vi "U01_4_MultipleClients.vi"() -> ()   [LabVIEW 2015]
panel:
  in  "Salir":bool
  out "data out 2":string
  in  "mode (standard) 2":T1(ring)
  out "error out":errorcluster
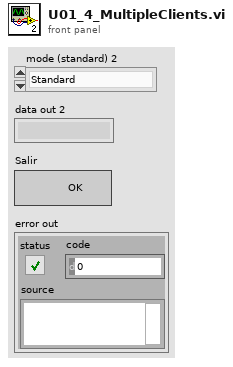
[diagram p1: front panel]
types:
  T1 = enum16{"Standard", "Buffered", "CRLF", "Immediate"}
  T2 = cluster{"connection ID":refnum<k5>, "service name":string, "port":u16}
  T3 = cluster{"Message":string, "ID":i32, "TCPCL":cluster{"connection ID":refnum<k5>, "service name":string, "port":u16}}
  T4 = cluster{string, "ID":i32, "TCPCL":cluster{"connection ID":refnum<k5>, "service name":string, "port":u16}}
  T5 = cluster{string, i32, "TCPCL":cluster{"connection ID":refnum<k5>, "service name":string, "port":u16}}
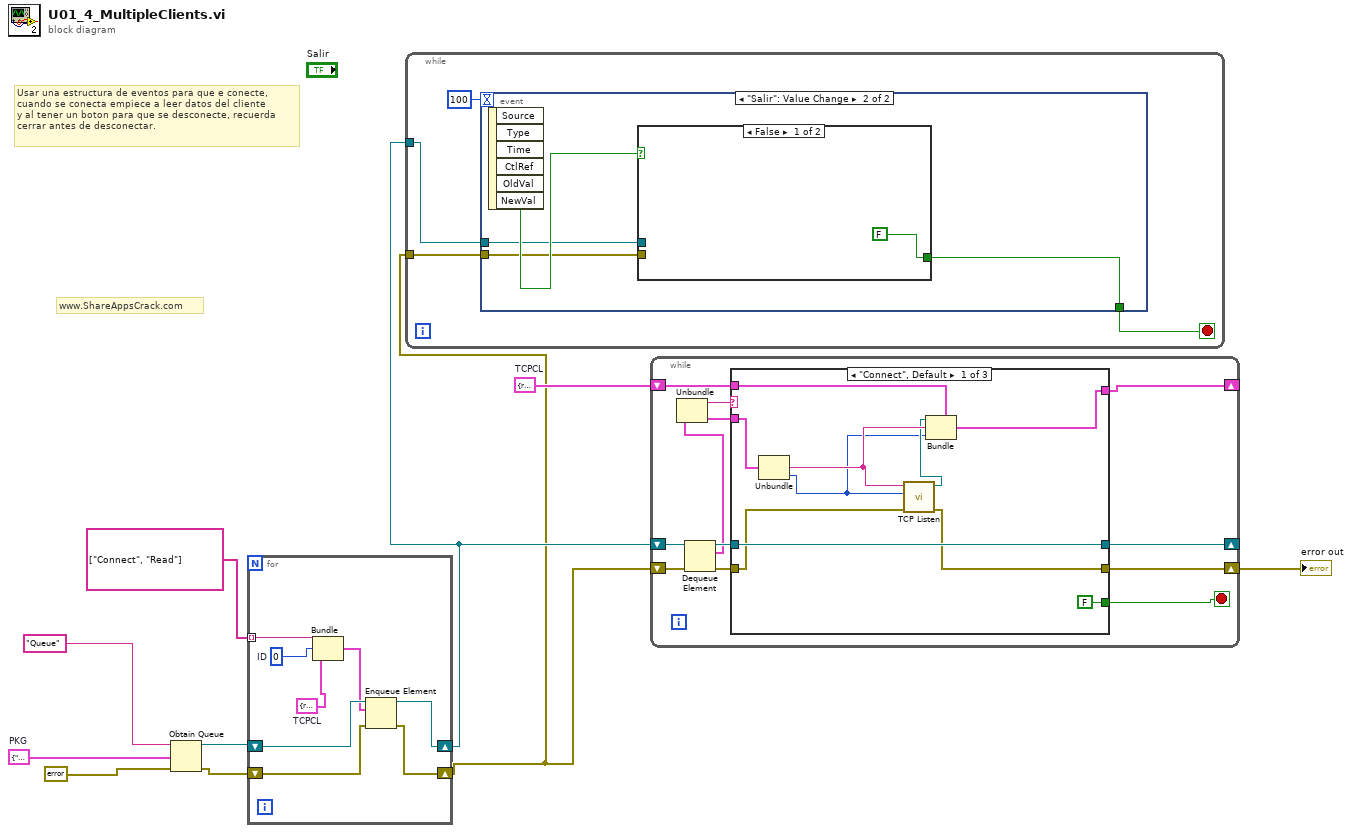
[diagram p0: block diagram]
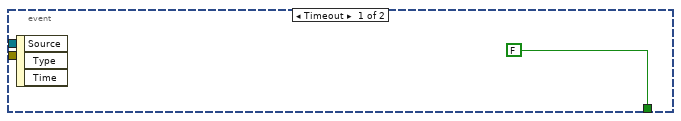
[diagram p2: hidden frame]
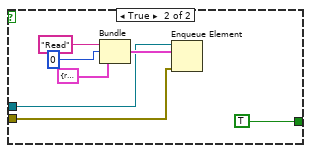
[diagram p3: hidden frame]
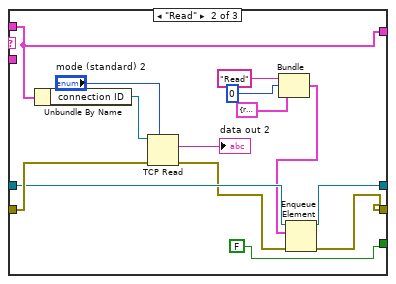
[diagram p4: hidden frame]
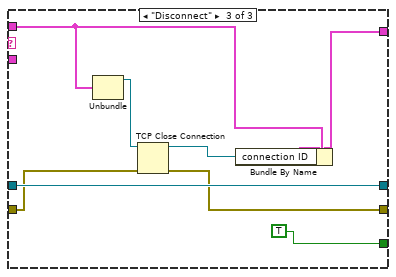
[diagram p5: hidden frame]
diagram:
  w3 = T2 {"connection ID"=refnum, "service name"="127.0.0.1", "port"=80}  # TCPCL
  w7 = T3 {"Message"="", "ID"=0, "TCPCL"={"connection ID"=refnum, "service name"="", "port"=0}}  # PKG
  # "Usar una estructura de eventos para que e conecte,\ncuando se conecta empiece a leer datos del cliente\ny al tener un boton para que se desconecte, recuerda \ncerrar antes de desconectar."
  # "www.ShareAppsCrack.com"
  n1 = Obtain Queue(name (unnamed)="Queue", element data type=w7, error in (no error)=errorcluster {"status"=FALSE, "code"=0, "source"=""}) -> (queue out=w6:refnum<queue>, error out=w5:errorcluster)  [unwired: 2 in, 1 out]
  n2 = for {
    shift-right: [w11] -> w2
    shift-left: w6 -> [w15]
    shift-right: [w12] -> w1
    shift-left: w5 -> [w13]
    tunnel: string[] ["Connect", "Read"] -> [w18] mode=indexing
    w16 = T2 {"connection ID"=refnum, "service name"="", "port"=0}  # TCPCL
    w17 = 0  # ID
    n3 = Bundle(w18, "ID"=w17, "TCPCL"=w16) -> (w14:T4)  [unwired: 1 in]
    n4 = Enqueue Element(queue=w15, element=w14, error in (no error)=w13) -> (queue out=w11:refnum<queue>, error out=w12:errorcluster)  [unwired: 1 in, 1 out]
  }
  n5 = while {
    tunnel: w2 -> [w21]
    tunnel: w1 -> [w20]
    stop <- w19 stop-if-true
    n6 = event shown="[1] \"Salir\": Value Change" {
      selector: _ -> [_ _]
      dyn-events: _ -> [_ _]
      timeout: 100 -> [_ _]
      tunnel: w21 -> [_ w26]
      tunnel: w20 -> [_ w25]
      tunnel: [FALSE w24] -> w19
      event Timeout {
        n7 = event-data() -> ()  [unwired: 1 in, 3 out]
      }
      event "Salir": Value Change {
        n8 = event-data() -> ("NewVal"=w27:bool)  [unwired: 1 in, 5 out]
        n9 = case shown="False" w27 {
          tunnel: w26 -> [_ w31]
          tunnel: w25 -> [_ w30]
          tunnel: [FALSE TRUE] -> w24
          frame False {
          }
          frame True {
            n10 = Bundle("Read", 0, "TCPCL"=T2 {"connection ID"=refnum, "service name"="127.0.0.1", "port"=80}) -> (w32:T5)  [unwired: 1 in]
            n11 = Enqueue Element(queue=w31, element=w32, error in (no error)=w30) -> ()  [unwired: 1 in, 3 out]
          }
        }
      }
    }
  }
  n12 = while {
    shift-right: [w46] -> w8
    shift-left: w1 -> [w42]
    shift-right: [w47] -> _
    shift-left: w2 -> [w44]
    shift-right: [w37] -> _
    shift-left: w3 -> [w36]
    stop <- w45 stop-if-true
    n13 = Dequeue Element(queue=w44, error in (no error)=w42) -> (queue out=w43:refnum<queue>, element=w40:T3, error out=w41:errorcluster)  [unwired: 1 in, 1 out]
    n14 = Unbundle(w40) -> ("Message"=w39:string, "TCPCL"=w38:T2)  [unwired: 1 out]
    n15 = case shown="\"Connect\", Default" w39 {
      tunnel: w41 -> [w56 w68 w78]
      tunnel: w43 -> [w57 w67 w79]
      tunnel: [w57 w66 w79] -> w47
      tunnel: [w55 w64 w77] -> w46
      tunnel: [FALSE ("status") FALSE TRUE] -> w45
      tunnel: w38 -> [w54 _ _]
      tunnel: [w48 w59 w74] -> w37
      tunnel: w36 -> [w52 w59 w75]
      frame "Connect", Default {
        n16 = Unbundle(w54) -> ("service name"=w51:string, "port"=w49:u16)  [unwired: 1 out]
        n17 = call <vilib>:"TCP Listen.vi"("error in (no error)"=w56, "port"=w49, "service name"=w51) -> ("error out"=w55:errorcluster, "connection ID"=w50:refnum<k5>)  [unwired: 4 in, 3 out]
        n18 = Bundle(cluster=w52, "connection ID"=w50, "service name"=w51, "port"=w49) -> (w48:T2)
      }
      frame "Read" {
        n19 = Unbundle By Name(w59) -> ("connection ID"=w71:refnum<k5>)
        n20 = TCP Read(connection ID=w71, error in (no error)=w68, 7:"mode (standard) 2") -> (data out=→"data out 2":string, error out=w65:errorcluster)  [unwired: 2 in, 1 out]
        n21 = Bundle("Read", 0, "TCPCL"=T2 {"connection ID"=refnum, "service name"="127.0.0.1", "port"=80}) -> (w60:T5)  [unwired: 1 in]
        n22 = Enqueue Element(queue=w67, element=w60, error in (no error)=w65) -> (queue out=w66:refnum<queue>, error out=w64:errorcluster)  [unwired: 1 in, 1 out]
      }
      frame "Disconnect" {
        n23 = Unbundle(w75) -> ("connection ID"=w76:refnum<k5>)  [unwired: 2 out]
        n24 = TCP Close Connection(connection ID=w76, error in (no error)=w78) -> (connection ID out=w73:refnum<k5>, error out=w77:errorcluster)  [unwired: 1 in]
        n25 = Bundle By Name(cluster=w75, "connection ID"=w73) -> (w74:T2)
      }
    }
  }
  "error out" <- w8
